vi "Write Owning Component's Product Name.vi"(8 "error in (no error)":errorcluster, 10 "Owning Component's Product Name":string, 11 "Export in":refnum<class "Export.lvclass">) -> (0 "error out":errorcluster, 3 "Export out":refnum<class "Export.lvclass">)   [LabVIEW 2017, in "CL_G3_VIComponentBuilder.lvlib" / "Export.lvclass"]
uses:
  Export.lvclass
  Export.lvclass/Export.ctl
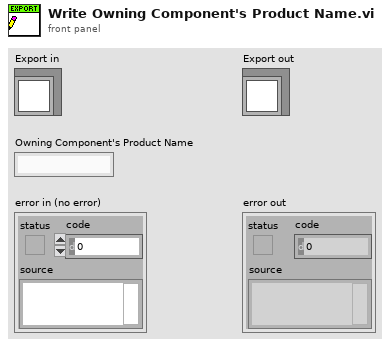
[diagram p1: front panel]
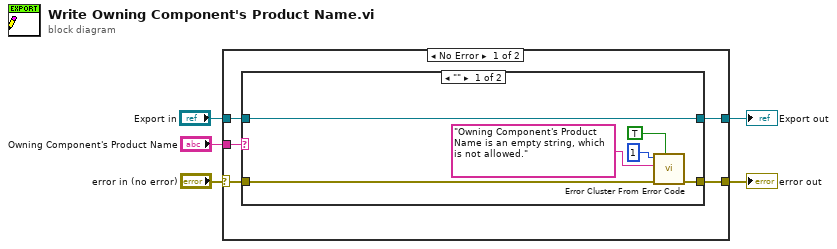
[diagram p0: block diagram]
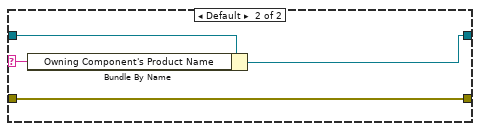
[diagram p2: hidden frame]
diagram:
  n1 = case shown="No Error" "error in (no error)" {
    selector: "error in (no error)" -> [w7 w21]
    tunnel: [w6 w21] -> w4
    tunnel: [w9 w22] -> w2
    tunnel: "Export in" -> [w10 w22]
    tunnel: "Owning Component's Product Name" -> [w8 _]
    frame No Error {
      n2 = case shown="\"\"" w8 {
        selector: w8 -> [_ w18]
        tunnel: w10 -> [w16 w20]
        tunnel: [w16 w19] -> w9
        tunnel: w7 -> [w12 w17]
        tunnel: [w11 w17] -> w6
        frame "" {
          n3 = call <vilib>:"Error Cluster From Error Code.vi"("show call chain? (False)"=TRUE, "error in (no error)"=w12, "error message (\"\")"="Owning Component's Product Name is an empty string, which is not allowed." ("error message (\"\")"), "error code (0)"=1) -> ("error out"=w11:errorcluster)  [unwired: 5 in]
        }
        frame Default {
          n4 = Bundle By Name(cluster=w20, "Owning Component's Product Name"=w18) -> (w19:refnum<class "Export.lvclass">)
        }
      }
    }
    frame Error {
    }
  }
  "error out" <- w4
  "Export out" <- w2
